vi "CC Script Check Telescope is Close Enough.vi"(10 "Current Pos":T1, 11 "Target Pos":T1) -> (1 "msg":string, 2 "In Range?":cluster{"RA":bool, "DEC":bool}, 3 "close enough":bool)   [LabVIEW 2021]
uses:
  typedefs/CC cluster RA and DEC.ctl
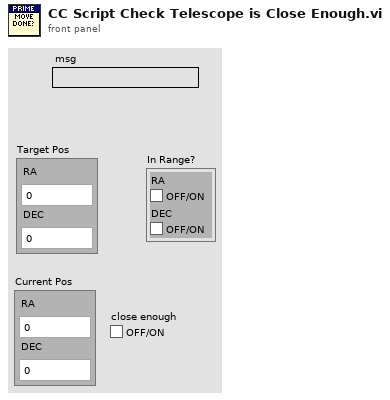
[diagram p1: front panel]
types:
  T1 = typedef "CC cluster RA and DEC.ctl" = cluster{"RA":dbl, "DEC":dbl}
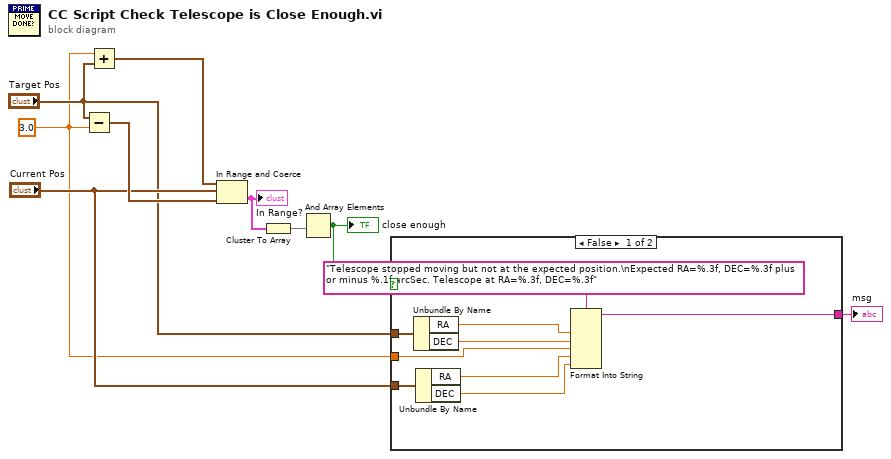
[diagram p0: block diagram]
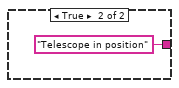
[diagram p2: hidden frame]
diagram:
  w1 = 3.0
  n1 = Subtract(x="Target Pos", y=w1) -> (x-y=w9:T1)
  n2 = Add(x=w1, y="Target Pos") -> (x+y=w6:T1)
  n3 = In Range and Coerce(upper limit=w6, x="Current Pos", lower limit=w9) -> (In Range?=w8:cluster{"RA":bool, "DEC":bool})  [unwired: 1 out]
  "In Range?" <- w8
  n4 = Cluster To Array(cluster=w8) -> (array=w7:bool[])
  n5 = And Array Elements(Boolean array=w7) -> (logical AND=w4:bool)
  "close enough" <- w4
  n6 = case shown="False" w4 {
    tunnel: "Target Pos" -> [w17 _]
    tunnel: "Current Pos" -> [w14 _]
    tunnel: [w11 "Telescope in position"] -> w3
    tunnel: w1 -> [w10 _]
    frame False {
      n7 = Unbundle By Name(w17) -> ("RA"=w16:dbl, "DEC"=w15:dbl)
      n8 = Unbundle By Name(w14) -> ("RA"=w13:dbl, "DEC"=w12:dbl)
      n9 = Format Into String(format string="Telescope stopped moving but not at the expected position.\nExpected RA=%.3f, DEC=%.3f plus or minus %.1f arcSec. Telescope at RA=%.3f, DEC=%.3f" ("Message"), w16, w15, w10, w13, w12) -> (resulting string=w11:string)  [unwired: 2 in, 1 out]
    }
    frame True {
    }
  }
  "msg" <- w3
